vi "ADO Recordset Move.vi"(0 "ADODB._Recordset In":refnum<k7>, 1 "NumRecords":i32, 5 "error in (no error)":errorcluster) -> (14 "ADODB._Recordset Out":refnum<k7>, 19 "error out":errorcluster)   [LabVIEW 2013]
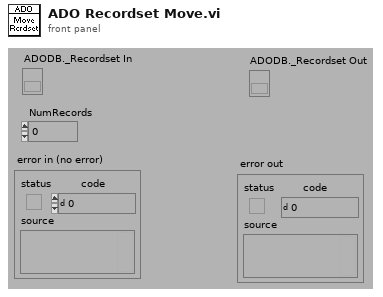
[diagram p1: front panel]
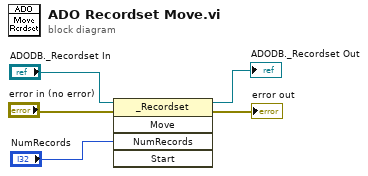
[diagram p0: block diagram]
diagram:
  n1 = invoke class="_Recordset" method="Move"(reference="ADODB._Recordset In", error in="error in (no error)", "NumRecords"="NumRecords") -> (reference out=→"ADODB._Recordset Out":refnum<k7>, error out=→"error out":errorcluster)  [unwired: 2 in, 3 out]
